vi "3458A Fetch from Digitizing Process.vi"(8 "error in":errorcluster, 11 "session in":T3 {"channels"."Range [Vpk]" min=0.0}) -> (0 "error out":errorcluster, 1 "aux data":T1, 2 "data packet":T2, 3 "session out":T3 {"channels"."Range [Vpk]" min=0.0}, 4 "fetching done?":bool)   [LabVIEW 2018, in "3458A Virtual Digitizer.lvlib"]
doc: "This VI fetches digitized samples from the digitizing processes initiated by 'Initiate Digitizing Process'. It checks the data queues of the particular channels and merges samples from the channels into 2D array whenever all channels return matching series of samples. Until all channels sends some samples to the queues it won't return data but also won't return error. When some of the digitizing processes exits with error or exits prematurely it will generate error. It will also generate error when fetching timeout occures. When processes seems to returnes unsynchronized data it will also generate error and terminate fetching. Called of this vi must keep checking flag 'valid?' in the 'data packet' and 'aux data'. When the flag is True the data must be checked/collected. When this VI returnes 'fetching done?' or error flag the caller shall not call the function again."
uses:
  3458A Virtual Digitizer.lvlib
  3458A Digitizer Session.ctl
  3458A Virtual Channel Config.ctl
  Counter/Counter Session.ctl
  Counter/Counter Type.ctl
  AWG/AWG Session.ctl
  AWG/AWG Type.ctl
  3458A Sync Mode.ctl
  3458A Idn Mode.ctl
  3458A Digitizing Low Levels/Configure/Sampling Mode.ctl
  3458A Digitizing Process Options.ctl
  3458A Data Packet.ctl
  3458A Aux Record Data.ctl
  3458A Digitizing Low Levels/Configure/Level Setup.ctl
  3458A Digitizing Low Levels/Configure/First Sample Trigger.ctl
  3458A Aperture Selection Mode.ctl
  <vilib>/Utility/error.llb/Error Cluster From Error Code.vi
  <vilib>/ErrorRing/Error Ring.xnode
  Counter/Counter.lvlib
  AWG/AWG.lvlib
  3458A Digitizing Low Levels/3458A Digitizing Low Levels.lvlib
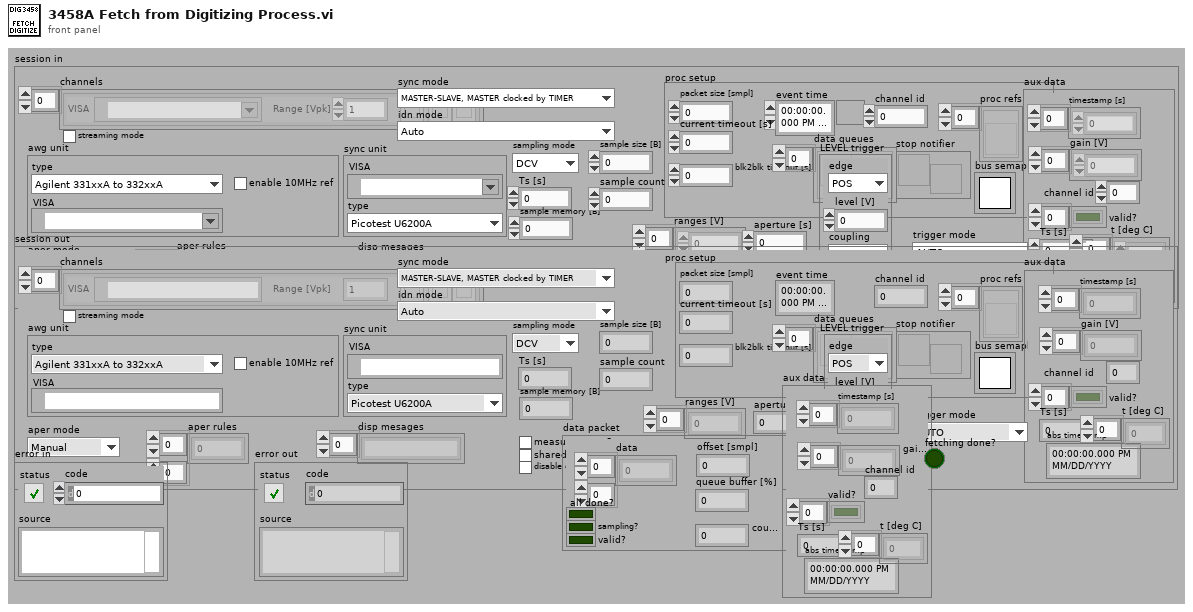
[diagram p1: front panel]
types:
  T1 = typedef "3458A Virtual Digitizer.lvlib/3458A Aux Record Data.ctl" = cluster{"channel id":i32, "valid?":bool[], "gain [V]":dbl[], "timestamp [s]":dbl[], "Ts [s]":dbl, "abs timestamp":timestamp, "t [deg C]":dbl[]}
  T2 = typedef "3458A Virtual Digitizer.lvlib/3458A Data Packet.ctl" = cluster{"data":i32[][], "offset [smpl]":i32, "count [smpl]":i32, "all done?":bool, "sampling?":bool, "queue buffer [%]":dbl, "valid?":bool}
  T3 = typedef "3458A Virtual Digitizer.lvlib/3458A Digitizer Session.ctl" = cluster{"channels":T4[], "sync unit":T5, "awg unit":T7, "sync mode":T9, "streaming mode":bool, "idn mode":T10, "sampling mode":T11, "Ts [s]":dbl, "sample memory [B]":i32, "proc setup":T12, "sample size [B]":i32, "sample count":i32, "aux data":T1, "ranges [V]":dbl[], "aperture [s]":dbl, "LEVEL trigger":T14, "trigger mode":T15, "measure temp.?":bool, "disp mesages":string[], "shared bus?":bool, "disable display?":bool, "aper mode":T16, "aper rules":dbl[][]}
  T4 = typedef "3458A Virtual Digitizer.lvlib/3458A Virtual Channel Config.ctl" = cluster{"VISA":refnum<visa-resource-name>, "Range [Vpk]":dbl, "btn clr":bool, "btn up":bool, "btn down":bool}
  T5 = typedef "Counter.lvlib/Counter Session.ctl" = cluster{"VISA":refnum<visa-resource-name>, "type":T6}
  T6 = typedef "Counter.lvlib/Counter Type.ctl" = enum16{"Picotest U6200A", "dummy"}
  T7 = typedef "AWG.lvlib/AWG Session.ctl" = cluster{"type":T8, "VISA":refnum<visa-resource-name>, "enable 10MHz ref":bool}
  T8 = typedef "AWG.lvlib/AWG Type.ctl" = enum16{"Agilent 331xxA to 332xxA", "Agilent 335xxA to 336xxA", "Tektronix AFG3101C", "dummy"}
  T9 = typedef "3458A Virtual Digitizer.lvlib/3458A Sync Mode.ctl" = enum16{"MASTER-SLAVE, MASTER clocked by TIMER", "MASTER-SLAVE, MASTER clocked by AWG", "ALL clocked by AWG", "MASTER-SLAVE, ALL clocked by TIMER", "ALL clocked by AWG with DFLL"}
  T10 = typedef "3458A Virtual Digitizer.lvlib/3458A Idn Mode.ctl" = enum16{"Auto", "Sequential (chn A, chn B, ...)", "From calibration string"}
  T11 = typedef "3458A Virtual Digitizer.lvlib/3458A Digitizing Low Levels.lvlib/Sampling Mode.ctl" = enum16{"DCV", "DSDC", "DSAC"}
  T12 = typedef "3458A Virtual Digitizer.lvlib/3458A Digitizing Process Options.ctl" = cluster{"channel id":i32, "packet size [smpl]":i32, "current timeout [s]":dbl, "blk2blk timeout [s]":dbl, "event time":timestamp, "stop notifier":refnum<notifier>, "data queues":refnum<queue>[], "proc refs":refnum<vi>[], "bus semaphore":T13}
  T13 = typedef "Semaphore RefNum" = refnum<k1>
  T14 = typedef "3458A Virtual Digitizer.lvlib/3458A Digitizing Low Levels.lvlib/Level Setup.ctl" = cluster{"edge":enum16{"POS", "NEG"}, "level [V]":dbl, "coupling":enum16{"DC", "AC"}}
  T15 = typedef "3458A Virtual Digitizer.lvlib/3458A Digitizing Low Levels.lvlib/First Sample Trigger.ctl" = enum16{"AUTO", "EXT", "SYN", "SGL", "HOLD", "LEVEL"}
  T16 = typedef "3458A Virtual Digitizer.lvlib/3458A Aperture Selection Mode.ctl" = enum16{"Manual", "Maximum", "Table"}
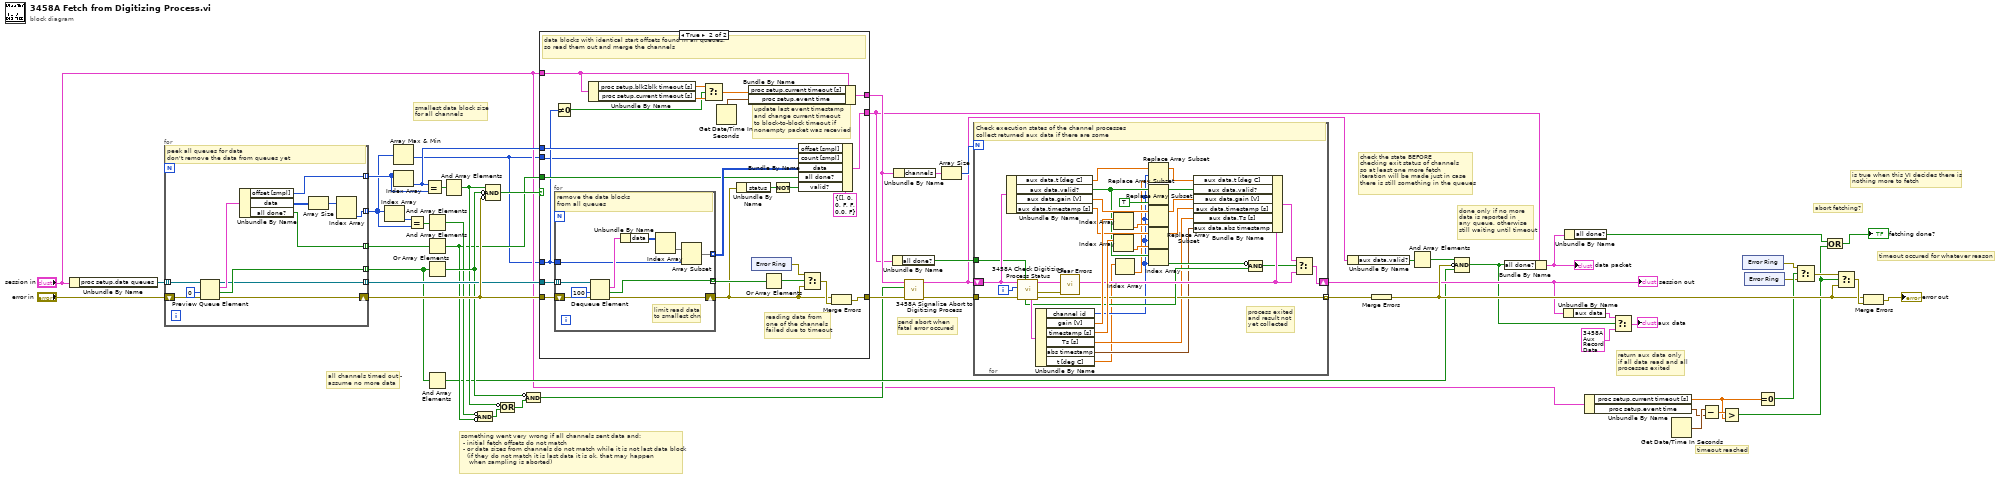
[diagram p0: block diagram]
diagram:
  # "abort fetching?"
  # "check the state BEFORE\nchecking exit status of channels \nso at least one more fetch\niteration will be made just in case \nthere is still something in the queues"
  # "return aux data only\nif all data read and all\nprocesses exited"
  # "done only if no more\ndata is reported in\nany queue, otherwise\nstill waiting until timeout"
  # "is true when this VI decides there is\nnothing more to fetch"
  # "timeout reached"
  # "send abort when\nfatal error occured"
  # "something went very wrong if all channels sent data and:\n - initial fetch offsets do not match\n - or data sizes from channels do not match while it is not last data block\n   (if they do not match it is last data it is ok, that may happen\n    when sampling is aborted)"
  # "all channels timed out -\nassume no more data"
  # "timeout occured for whatever reason"
  # "smallest data block size\nfor all channels"
  n1 = Unbundle By Name("session in") -> ("proc setup.data queues"=w26:refnum<queue>[])
  n2 = for {
    tunnel: w26 -> [w65] mode=indexing
    tunnel: [w62] -> w39 mode=indexing
    tunnel: [w55] -> w49 mode=indexing
    tunnel: [w58] -> w53 mode=indexing
    shift-right: [w63] -> w47
    shift-left: "error in" -> [w66]
    tunnel: [w57] -> w48 mode=indexing
    tunnel: [w56] -> w46 mode=indexing
    # "peek all queues for data\ndon't remove the data from queues yet"
    n3 = Preview Queue Element(queue=w65, timeout in ms (-1)=0, error in (no error)=w66) -> (queue out=w56:refnum<queue>, element=w61:T2, timed out?=w62:bool, error out=w63:errorcluster)
    n4 = Unbundle By Name(w61) -> ("offset [smpl]"=w58:i32, "data"=w60:i32[][], "all done?"=w57:bool)
    n5 = Array Size(array=w60) -> (size(s)=w59:i32[])
    n6 = Index Array(array=w59) -> (element #2=w55:i32)  [unwired: 2 in, 1 out]
  }
  n7 = Index Array(array=w49) -> (element=w50:i32)  [unwired: 1 in]
  n8 = Array Max & Min(array=w49) -> (min value=w1:i32)  [unwired: 3 out]
  n9 = Index Array(array=w53) -> (element=w44:i32)  [unwired: 1 in]
  n10 = Equal?(x=w50, y=w49) -> (x = y?=w51:bool[])
  n11 = Equal?(x=w44, y=w53) -> (x = y?=w52:bool[])
  n12 = And Array Elements(Boolean array=w51) -> (logical AND=w34:bool)
  n13 = And Array Elements(Boolean array=w48) -> (logical AND=w33:bool)
  n14 = Or Array Elements(Boolean array=w39) -> (logical OR=w38:bool)
  n15 = And Array Elements(Boolean array=w39) -> (logical AND=w18:bool)
  n16 = And Array Elements(Boolean array=w52) -> (logical AND=w36:bool)
  n17 = Compound Arithmetic op=AND(invert w34, invert w33) -> (w35:bool)
  n18 = Compound Arithmetic op=AND(w36, invert w38, invert w47) -> (w45:bool)
  n19 = Compound Arithmetic op=OR(invert w36, w35) -> (w37:bool)
  n20 = Compound Arithmetic op=AND(invert w38, w37) -> (w3:bool)
  n21 = case shown="True" w45 {
    tunnel: w47 -> [w68 w92]
    tunnel: w46 -> [_ w91]
    tunnel: [w68 w86] -> w32
    tunnel: w1 -> [_ w79]
    tunnel: w33 -> [_ w83]
    tunnel: w44 -> [_ w82]
    tunnel: [_ w81] -> w16
    tunnel: "session in" -> [w67 w77]
    tunnel: [w67 w80] -> w30
    tunnel: w1 -> [_ w69]
    frame False {
      # "error or read data offsets of from various channels do not match"
    }
    frame True {
      # "update last event timestamp\nand change current timeout\nto block-to-block timeout if\nnonempty packet was recevied"
      # "reading data from\none of the channels\nfailed due to timeout"
      # "data blocks with identical start offsets found in all queues,\nso read them out and merge the channels"
      n22 = Not Equal To 0?(x=w79) -> (x != 0?=w74:bool)
      n23 = for {
        tunnel: w91 -> [w106] mode=indexing
        tunnel: [w103] -> w90 mode=indexing
        shift-right: [w104] -> w72
        shift-left: w92 -> [w107]
        tunnel: w79 -> [w101]
        tunnel: [w99] -> w84 mode=indexing
        # "limit read data\nto smallest chn"
        # "remove the data blocks\nfrom all queues"
        n24 = Dequeue Element(queue=w106, timeout in ms (-1)=100, error in (no error)=w107) -> (element=w102:T2, timed out?=w103:bool, error out=w104:errorcluster)  [unwired: 1 out]
        n25 = Unbundle By Name(w102) -> ("data"=w100:i32[][])
        n26 = Index Array(array=w100) -> (element=w98:i32[])  [unwired: 2 in]
        n27 = Array Subset(array=w98, length=w101) -> (w99:i32[])  [unwired: 1 in]
      }
      n28 = Unbundle By Name(w77) -> ("proc setup.blk2blk timeout [s]"=w76:dbl, "proc setup.current timeout [s]"=w75:dbl)
      n29 = Select(t=w76, s=w74, f=w75) -> (s? t:f=w73:dbl)
      n30 = Get Date/Time In Seconds() -> (seconds since 1Jan1904=w78:timestamp)
      n31 = Unbundle By Name(w72) -> ("status"=w71:bool)
      n32 = Bundle By Name(cluster=w77, "proc setup.current timeout [s]"=w73, "proc setup.event time"=w78) -> (w80:T3)
      n33 = xnode "Error Ring"() -> ("error out"=w88:errorcluster)
      n34 = Or Array Elements(Boolean array=w90) -> (logical OR=w89:bool)
      n35 = Not(x=w71) -> (.not. x?=w70:bool)
      n36 = Bundle By Name(cluster=T2 {"data"=[], "offset [smpl]"=0, "count [smpl]"=0, "all done?"=FALSE, "sampling?"=FALSE, "queue buffer [%]"=0.0, "valid?"=FALSE} ("niScope packet"), "offset [smpl]"=w82, "count [smpl]"=w69, "data"=w84, "all done?"=w83, "valid?"=w70) -> (w81:T2)
      n37 = Select(t=w88, s=w89, f=w72) -> (s? t:f=w87:errorcluster)
      n38 = Merge Errors(w72, w87) -> (w86:errorcluster)
    }
  }
  n39 = Unbundle By Name(w16) -> ("all done?"=w15:bool)
  n40 = Unbundle By Name(w30) -> ("channels"=w43:T4[])
  n41 = call "3458A Signalize Abort to Digitizing Process.vi"("error in"=w32, "send abort signal? (True)"=w3, "session in"=w30) -> ("error out (copy)"=w31:errorcluster, "session out"=w12:T3)  [unwired: 7 in]
  n42 = Array Size(array=w43) -> (size(s)=w40:i32)
  n43 = for {
    N: w40 -> [_]
    tunnel: w31 -> [w138]
    tunnel: [w116] -> w42 mode=indexing
    shift-right: [w118] -> w22
    shift-left: w12 -> [w128]
    tunnel: w15 -> [w117]
    i -> [w137]
    # "process exited\nand result not \nyet collected"
    # "Check execution states of the channel processes\ncollect returned aux data if there are some"
    n44 = Unbundle By Name(w128) -> ("aux data.t [deg C]"=w110:dbl[], "aux data.valid?"=w122:bool[], "aux data.gain [V]"=w134:dbl[], "aux data.timestamp [s]"=w129:dbl[])
    n45 = call "3458A Check Digitizing Process Status.vi"("wait for exit (False)"=w117, "error in"=w138, "channel id"=w137, "digitizer session in"=w128) -> ("error out"=w116:errorcluster, "proc error out"=w115:errorcluster, "digitizer session out"=w124:T3, "aux data out"=w136:T1, "aux data valid?"=w121:bool)  [unwired: 2 in, 1 out]
    n46 = Unbundle By Name(w136) -> ("channel id"=w111:i32, "gain [V]"=w133:dbl[], "timestamp [s]"=w131:dbl[], "Ts [s]"=w114:dbl, "abs timestamp"=w113:timestamp, "t [deg C]"=w109:dbl[])
    n47 = call <vilib>:"Clear Errors.vi"("error in (no error)"=w115) -> ()  [unwired: 5 in, 2 out]
    n48 = Index Array(array=w133) -> (element=w132:dbl)  [unwired: 1 in]
    n49 = Index Array(array=w131) -> (element=w130:dbl)  [unwired: 1 in]
    n50 = Index Array(array=w109) -> (element=w108:dbl)  [unwired: 1 in]
    n51 = Replace Array Subset(array=w110, new element=w108, index=w111) -> (w112:dbl[])
    n52 = Replace Array Subset(array=w122, new element=TRUE ("new element/subarray"), index=w111) -> (w127:bool[])
    n53 = Replace Array Subset(array=w134, new element=w132, index=w111) -> (w126:dbl[])
    n54 = Replace Array Subset(array=w129, new element=w130, index=w111) -> (w123:dbl[])
    n55 = Index Array(array=w122, index=w111) -> (element=w120:bool)
    n56 = Bundle By Name(cluster=w124, "aux data.t [deg C]"=w112, "aux data.valid?"=w127, "aux data.gain [V]"=w126, "aux data.timestamp [s]"=w123, "aux data.Ts [s]"=w114, "aux data.abs timestamp"=w113) -> (w125:T3)
    n57 = Compound Arithmetic op=AND(invert w120, w121) -> (w119:bool)
    n58 = Select(t=w125, s=w119, f=w124) -> (s? t:f=w118:T3)
  }
  "session out" <- w22
  n59 = Unbundle By Name(w12) -> ("aux data.valid?"=w24:bool[])
  n60 = Merge Errors(w42) -> (w28:errorcluster)
  n61 = And Array Elements(Boolean array=w24) -> (logical AND=w23:bool)
  n62 = Compound Arithmetic op=AND(w23, invert w28, w18) -> (w17:bool)
  n63 = Bundle By Name(cluster=w16, "all done?"=w17) -> (w27:T2)
  "data packet" <- w27
  n64 = Unbundle By Name(w22) -> ("aux data"=w21:T1)
  n65 = Unbundle By Name(w27) -> ("all done?"=w5:bool)
  n66 = Unbundle By Name("session in") -> ("proc setup.current timeout [s]"=w10:dbl, "proc setup.event time"=w13:timestamp)
  n67 = Select(t=w21, s=w17, f=T1 {"channel id"=0, "valid?"=[], "gain [V]"=[], "timestamp [s]"=[], "Ts [s]"=0.0, "abs timestamp"=timestamp(0 s since 1904-01-01), "t [deg C]"=[]}) -> (s? t:f=→"aux data":T1)
  n68 = Get Date/Time In Seconds() -> (seconds since 1Jan1904=w14:timestamp)
  n69 = Subtract(x=w14, y=w13) -> (x-y=w29:dbl)
  n70 = Greater?(x=w29, y=w10) -> (0:w6:bool)
  n71 = xnode "Error Ring"() -> ("error out"=w7:errorcluster)
  n72 = xnode "Error Ring"() -> ("error out"=w8:errorcluster)
  n73 = Equal To 0?(x=w10) -> (x = 0?=w9:bool)
  n74 = Select(t=w7, s=w9, f=w8) -> (s? t:f=w11:errorcluster)
  n75 = Compound Arithmetic op=OR(w5, w6) -> (→"fetching done?":bool)
  n76 = Select(t=w11, s=w6, f=w28) -> (s? t:f=w41:errorcluster)
  n77 = Merge Errors(w28, w41) -> (→"error out":errorcluster)
